vi "DrawArrow.vi"(1 "Pen Style":T2={"Width"=1, "Style"=enum."Solid"}, 2 "Arena Pixel Dim":i32[](array[numeric])=[1000, 512], 3 "Color":u32(colorbox), 4 "Length (m)":dbl=0.5 format="%#_13g", 5 "Vector (m)":T1={"x"=1.0, "y"=1.0, "angle"=1.0}, 6 "picture":picture) -> (0 "new picture":picture)   [LabVIEW 2015, in "MissionControl2017.lvlib"]
uses:
  Vector.ctl
  MissionControl2017.lvlib
  Navigation2017.lvlib
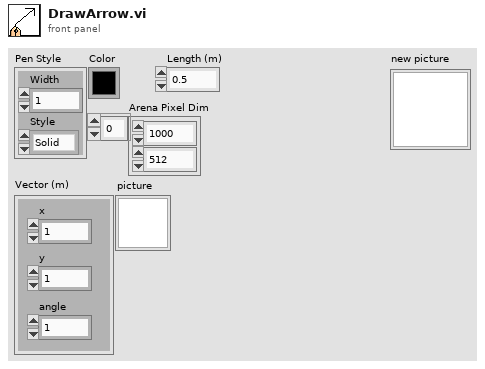
[diagram p1: front panel]
types:
  T1 = typedef "Navigation2017.lvlib/Vector.ctl" = cluster{"x":dbl, "y":dbl, "angle":dbl}
  T2 = cluster{"Width":u16, "Style":enum32{"Solid", "Dash", "Dot", "DashDot", "DashDotDot"}}
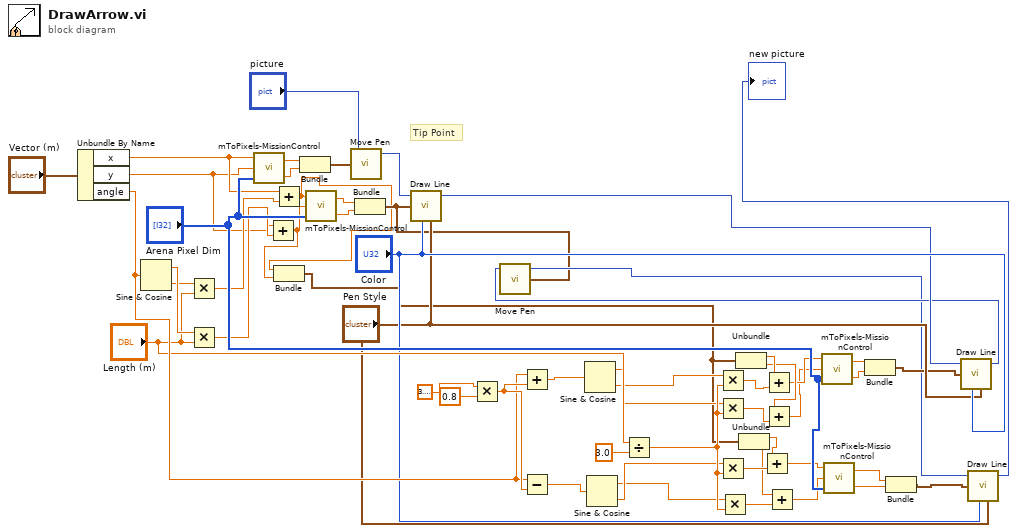
[diagram p0: block diagram]
diagram:
  # "Tip Point"
  n1 = Unbundle By Name("Vector (m)") -> ("x"=w5:dbl, "y"=w4:dbl, "angle"=w45:dbl)
  n2 = Sine & Cosine(0:w45) -> (1:w56:dbl, 2:w55:dbl)
  n3 = Multiply(x=w55, y="Length (m)") -> (x*y=w6:dbl)
  n4 = Multiply(x=w56, y="Length (m)") -> (x*y=w7:dbl)
  n5 = call "mToPixels-MissionControl.vi"("Arena Pixel Dim"="Arena Pixel Dim", "y (m)"=w4, "x (m)"=w5) -> ("y (pixels)"=w50:dbl, "x (pixels)"=w51:dbl)
  n6 = Add(x=w4, y=w7) -> (x+y=w1:dbl)
  n7 = Add(x=w5, y=w6) -> (x+y=w2:dbl)
  n8 = Bundle(w2, w1) -> (w3:cluster{dbl, dbl})  [unwired: 1 in]
  n9 = Bundle("x (pixels)"=w51, "y (pixels)"=w50) -> (w54:cluster{"x (pixels)":dbl, "y (pixels)":dbl})  [unwired: 1 in]
  n10 = call "mToPixels-MissionControl.vi"("Arena Pixel Dim"="Arena Pixel Dim", "y (m)"=w1, "x (m)"=w2) -> ("y (pixels)"=w8:dbl, "x (pixels)"=w9:dbl)
  n11 = call <vilib>:"Move Pen.vi"("new position"=w54, "picture"="picture") -> ("new picture"=w53:picture)  [unwired: 3 in]
  n12 = Bundle("x (pixels)"=w9, "y (pixels)"=w8) -> (w16:cluster{"x (pixels)":dbl, "y (pixels)":dbl})  [unwired: 1 in]
  n13 = call <vilib>:"Draw Line.vi"("picture"=w53, "end point"=w16, "color(black)"="Color", "pen"="Pen Style") -> ("new picture"=w25:picture)  [unwired: 5 in]
  n14 = Multiply(x=3.141592653589793, y=0.8) -> (x*y=w46:dbl)
  n15 = Add(x=w45, y=w46) -> (x+y=w44:dbl)
  n16 = Subtract(x=w45, y=w46) -> (x-y=w43:dbl)
  n17 = Sine & Cosine(0:w44) -> (1:w27:dbl, 2:w26:dbl)
  n18 = Sine & Cosine(0:w43) -> (1:w28:dbl, 2:w29:dbl)
  n19 = Divide(x="Length (m)", y=3.0) -> (x/y=w30:dbl)
  n20 = Multiply(x=w26, y=w30) -> (x*y=w19:dbl)
  n21 = Multiply(x=w27, y=w30) -> (x*y=w20:dbl)
  n22 = Multiply(x=w29, y=w30) -> (x*y=w21:dbl)
  n23 = Multiply(x=w28, y=w30) -> (x*y=w22:dbl)
  n24 = Unbundle(w3) -> (w18:dbl, w17:dbl)
  n25 = Unbundle(w3) -> (w15:dbl, w14:dbl)
  n26 = Add(x=w15, y=w21) -> (x+y=w11:dbl)
  n27 = Add(x=w18, y=w19) -> (x+y=w13:dbl)
  n28 = Add(x=w17, y=w20) -> (x+y=w12:dbl)
  n29 = Add(x=w14, y=w22) -> (x+y=w10:dbl)
  n30 = call "mToPixels-MissionControl.vi"("Arena Pixel Dim"="Arena Pixel Dim", "y (m)"=w12, "x (m)"=w13) -> ("y (pixels)"=w35:dbl, "x (pixels)"=w36:dbl)
  n31 = call "mToPixels-MissionControl.vi"("Arena Pixel Dim"="Arena Pixel Dim", "y (m)"=w10, "x (m)"=w11) -> ("y (pixels)"=w31:dbl, "x (pixels)"=w32:dbl)
  n32 = Bundle("x (pixels)"=w36, "y (pixels)"=w35) -> (w34:cluster{"x (pixels)":dbl, "y (pixels)":dbl})  [unwired: 1 in]
  n33 = Bundle("x (pixels)"=w32, "y (pixels)"=w31) -> (w33:cluster{"x (pixels)":dbl, "y (pixels)":dbl})  [unwired: 1 in]
  n34 = call <vilib>:"Draw Line.vi"("picture"=w25, "end point"=w34, "color(black)"="Color", "pen"="Pen Style") -> ("new picture"=w24:picture)  [unwired: 5 in]
  n35 = call <vilib>:"Move Pen.vi"("new position"=w16, "picture"=w24) -> ("new picture"=w23:picture)  [unwired: 3 in]
  n36 = call <vilib>:"Draw Line.vi"("picture"=w23, "end point"=w33, "color(black)"="Color", "pen"="Pen Style") -> ("new picture"=→"new picture":picture)  [unwired: 5 in]
